vi "csuTestResponsiveness.vi"() -> ()   [LabVIEW 2017]
panel:
  out "close":bool
  out "open":bool
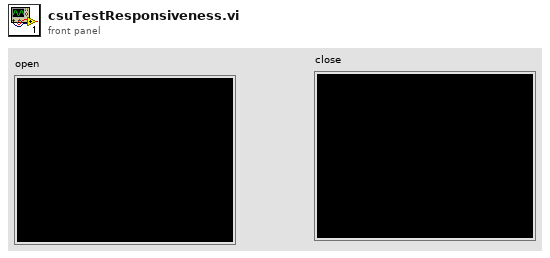
[diagram p1: front panel]
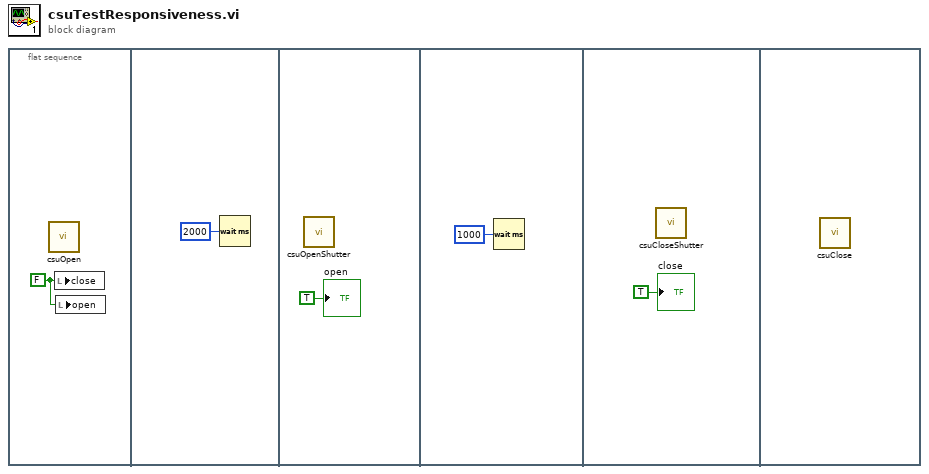
[diagram p0: block diagram]
diagram:
  n1 = flat-sequence {
    frame #0 {
      w1 = FALSE ("close")
      n2 = call "csuOpen.vi"() -> ()  [unwired: 14 in, 2 out]
      n3 = local write "close"(w1) -> ()
      n4 = local write "open"(w1) -> ()
    }
    frame #1 {
      n5 = Wait (ms)(milliseconds to wait=u32 2000) -> ()  [unwired: 1 out]
    }
    frame #2 {
      n6 = call "csuOpenShutter.vi"() -> ()  [unwired: 16 in]
      "open" <- TRUE ("open")
    }
    frame #3 {
      n7 = Wait (ms)(milliseconds to wait=u32 1000) -> ()  [unwired: 1 out]
    }
    frame #4 {
      n8 = call "csuCloseShutter.vi"() -> ()  [unwired: 16 in]
      "close" <- TRUE ("open")
    }
    frame #5 {
      n9 = call "csuClose.vi"() -> ()  [unwired: 12 in]
    }
  }
